vi "SetParam.vi"(8 "error in (no error)":errorcluster caption="entrée d'erreur (pas d'erreur)", 10 "SparseRandomProjection":T1={"n_components"="auto", "density"="auto", "eps"=0.1, "dense_output"=FALSE, "random_state"=-1} {"random_state" min=-1; "eps" min=0.0}, 11 "SparseRandomProjection.lvclass":refnum<class "SparseRandomProjection.lvclass">) -> (0 "error out":errorcluster caption="sortie d'erreur", 3 "SparseRandomProjection.lvclass":refnum<class "SparseRandomProjection.lvclass">)   [LabVIEW 2020, in "SparseRandomProjection.lvclass"]
doc: "Set Parameters"
uses:
  SparseRandomProjection.lvclass
  SparseRandomProjection.lvclass/SparseRandomProjection.ctl
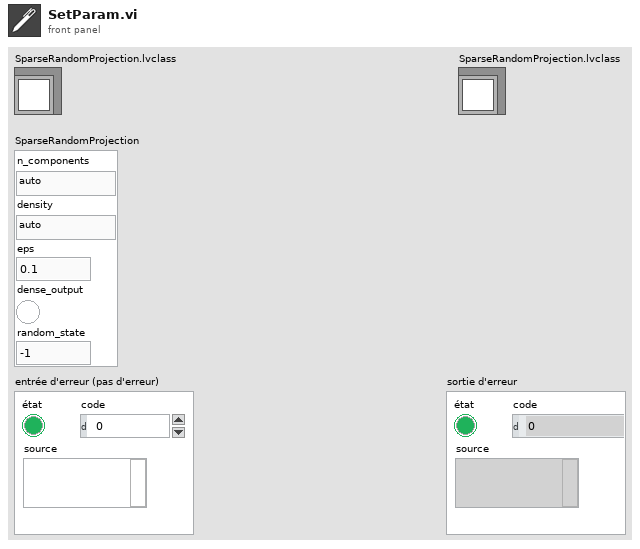
[diagram p1: front panel]
types:
  T1 = cluster{"n_components":string, "density":string, "eps":dbl, "dense_output":bool, "random_state":i32}
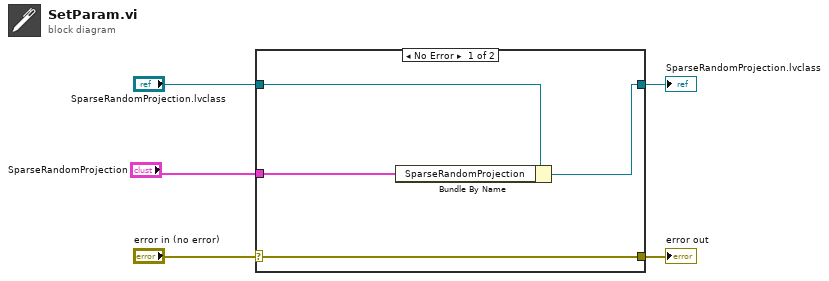
[diagram p0: block diagram]
diagram:
  n1 = case shown="No Error" "error in (no error)" {
    selector: "error in (no error)" -> [w9 w10]
    tunnel: [w9 w10] -> w4
    tunnel: [w7 w11] -> w2
    tunnel: "SparseRandomProjection.lvclass" -> [w8 w11]
    tunnel: "SparseRandomProjection" -> [w6 _]
    frame No Error {
      n2 = Bundle By Name(cluster=w8, "SparseRandomProjection"=w6) -> (w7:refnum<class "SparseRandomProjection.lvclass">)
    }
    frame Error {
    }
  }
  "error out" <- w4
  "SparseRandomProjection.lvclass" <- w2
